vi "AutoTrackRobot.vi"(11 "StartCoordinates":dbl[](array[numeric])) -> (3 "Coordinates":dbl[](array[numeric]))   [LabVIEW 2018]
uses:
  Swerve/SwerveGlobals.vi
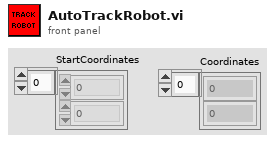
[diagram p1: front panel]
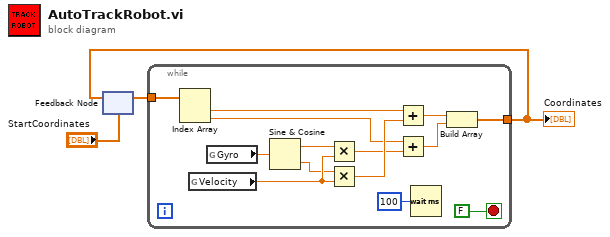
[diagram p0: block diagram]
diagram:
  n1 = feedback #1("StartCoordinates") -> (w3:dbl[])
  n2 = while {
    tunnel: w3 -> [w15]
    tunnel: [w5] -> w1
    stop <- FALSE stop-if-true
    n3 = Index Array(array=w15) -> (element #1=w14:dbl, element #2=w9:dbl)  [unwired: 2 in]
    n4 = global read "SwerveGlobals.vi" "Velocity"() -> (w12:dbl)
    n5 = global read "SwerveGlobals.vi" "Gyro"() -> (w16:dbl)
    n6 = Sine & Cosine(0:w16) -> (1:w13:dbl, 2:w11:dbl)
    n7 = Multiply(x=w13, y=w12) -> (x*y=w8:dbl)
    n8 = Multiply(x=w11, y=w12) -> (x*y=w10:dbl)
    n9 = Add(x=w14, y=w10) -> (x+y=w7:dbl)
    n10 = Add(x=w9, y=w8) -> (x+y=w6:dbl)
    n11 = Wait (ms)(milliseconds to wait=u32 100) -> ()  [unwired: 1 out]
    n12 = Build Array(w7, w6) -> (w5:dbl[])
  }
  "Coordinates" <- w1
  n13 = feedback-in #1(w1) -> ()
